vi "HW_6p1_Task2_gamagetd.vi"() -> ()   [LabVIEW 2016]
panel:
  out "Average Tem":dbl
  out "Number above 250":dbl
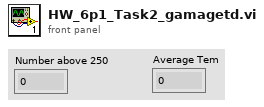
[diagram p1: front panel]
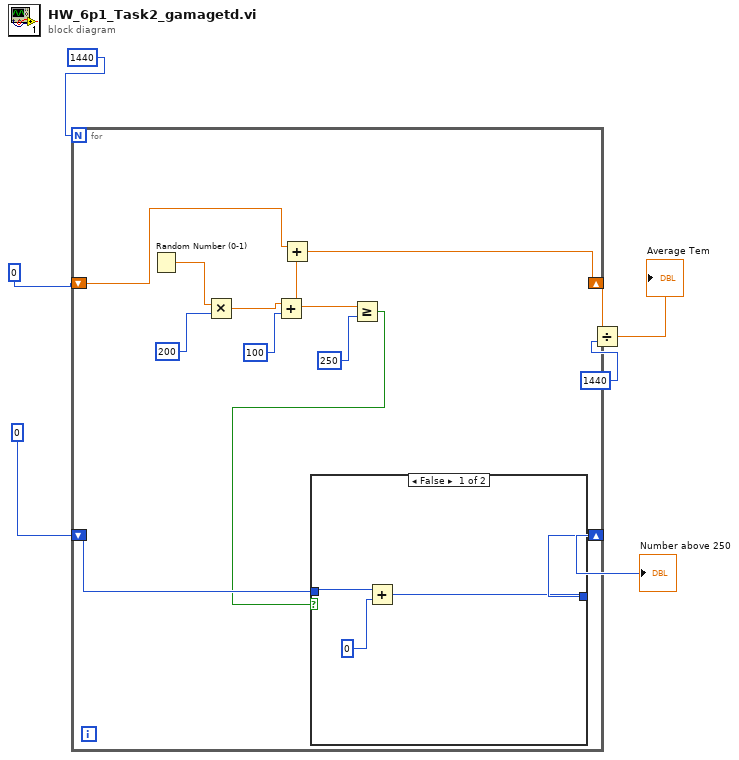
[diagram p0: block diagram]
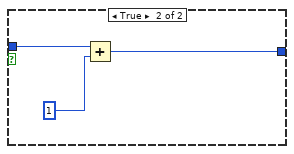
[diagram p2: hidden frame]
diagram:
  n1 = for {
    N: 1440 -> [_]
    shift-right: [w12] -> w5
    shift-left: 0 -> [w13]
    shift-right: [w9] -> w3
    shift-left: 0 -> [w11]
    n2 = Random Number (0-1)() -> (number: 0 to 1=w18:dbl)
    n3 = Multiply(x=w18, y=200) -> (x*y=w16:dbl)
    n4 = Add(x=w16, y=100) -> (x+y=w10:dbl)
    n5 = Add(x=w11, y=w10) -> (x+y=w9:dbl)
    n6 = Greater Or Equal?(x=w10, y=250) -> (x >= y?=w8:bool)
    n7 = case shown="False" w8 {
      tunnel: w13 -> [w21 w24]
      tunnel: [w19 w22] -> w12
      frame False {
        n8 = Add(x=w21, y=0) -> (x+y=w19:i32)
      }
      frame True {
        n9 = Add(x=w24, y=1) -> (x+y=w22:i32)
      }
    }
  }
  "Number above 250" <- w5
  n10 = Divide(x=w3, y=1440) -> (x/y=→"Average Tem":dbl)
